vi "Obtain Queue.vi"(8 "error in (no error)":errorcluster, 10 "Queue Name (in)":string, 11 "Messaging in":refnum<class "Messaging.lvclass">) -> (0 "error out":errorcluster, 3 "Messaging out":refnum<class "Messaging.lvclass">)   [LabVIEW 2023, in "MessagingModule.lvlib" / "Messaging.lvclass"]
uses:
  Messaging.lvclass
  Messaging.lvclass/Messaging.ctl
  Msg/Msg.Data.ctl
  MessagingModule.lvlib
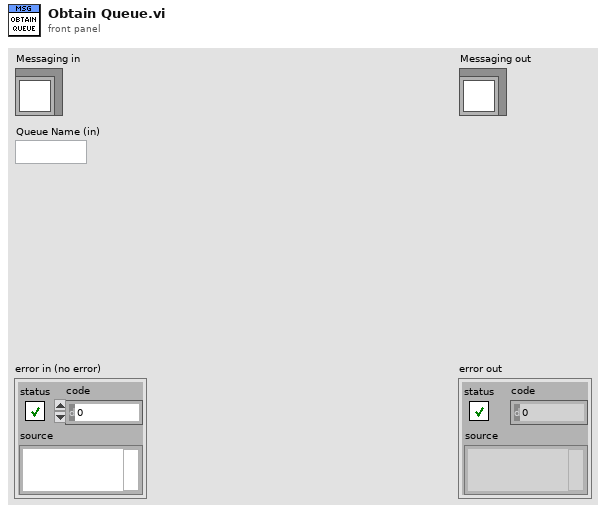
[diagram p1: front panel]
types:
  T1 = typedef "MessagingModule.lvlib/Msg.Data.ctl" = cluster{"Message":string, "Data":variant}
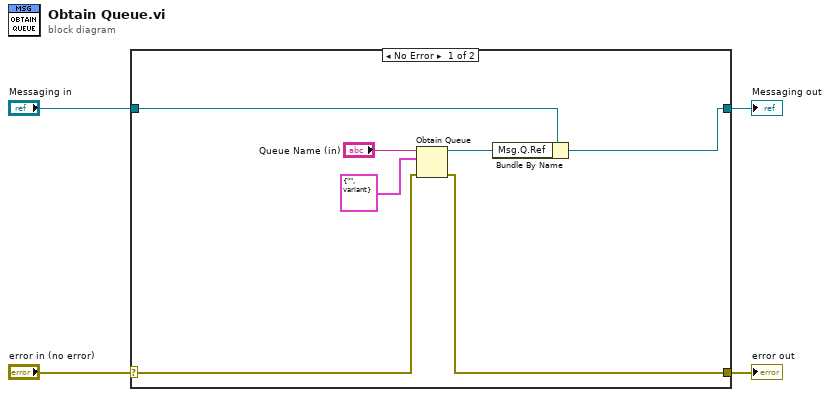
[diagram p0: block diagram]
diagram:
  n1 = case shown="No Error" "error in (no error)" {
    selector: "error in (no error)" -> [w9 w13]
    tunnel: [w8 w13] -> w3
    tunnel: [w5 w12] -> w1
    tunnel: "Messaging in" -> [w7 w12]
    frame No Error {
      n2 = Obtain Queue(name (unnamed)="Queue Name (in)", element data type=T1 {"Message"="", "Data"=variant} ("Msg.Q.Data"), error in (no error)=w9) -> (queue out=w6:refnum<queue>, error out=w8:errorcluster)  [unwired: 2 in, 1 out]
      n3 = Bundle By Name(cluster=w7, "Msg.Q.Ref"=w6) -> (w5:refnum<class "Messaging.lvclass">)
    }
    frame Error {
    }
  }
  "error out" <- w3
  "Messaging out" <- w1
